vi "ClearAll.vi"(8 "Error In":errorcluster, 11 "CommunicationRefs":T1) -> (0 "error out":errorcluster)   [LabVIEW 2015]
uses:
  TypeDefs/CommunicationRefs.ctl
  TypeDefs/MessageCluster.ctl
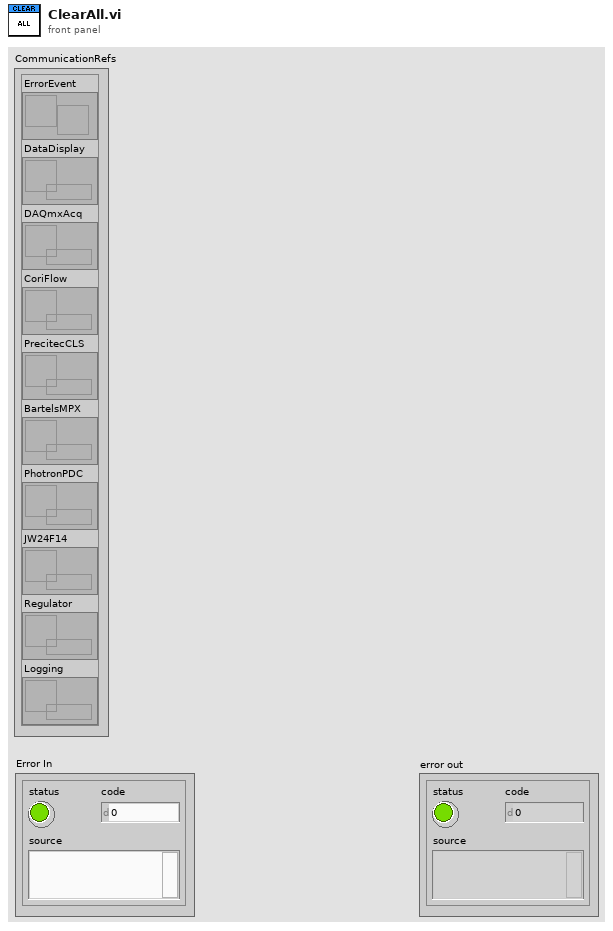
[diagram p1: front panel]
types:
  T1 = typedef "CommunicationRefs.ctl" = cluster{"ErrorEvent":refnum<user-event>, "DataDisplay":refnum<queue>, "DAQmxAcq":refnum<queue>, "CoriFlow":refnum<queue>, "PrecitecCLS":refnum<queue>, "BartelsMPX":refnum<queue>, "PhotronPDC":refnum<queue>, "JW24F14":refnum<queue>, "Regulator":refnum<queue>, "Logging":refnum<queue>}
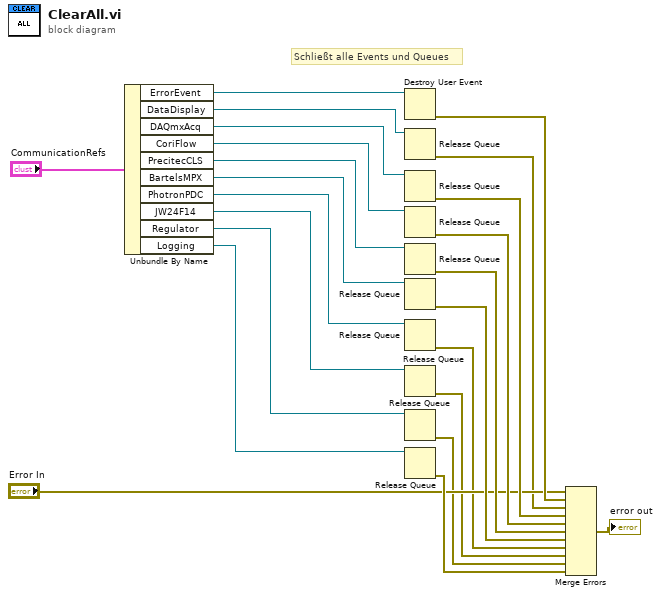
[diagram p0: block diagram]
diagram:
  # "Schließt alle Events und Queues"
  n1 = Unbundle By Name("CommunicationRefs") -> ("ErrorEvent"=w22:refnum<user-event>, "DataDisplay"=w8:refnum<queue>, "DAQmxAcq"=w20:refnum<queue>, "CoriFlow"=w19:refnum<queue>, "PrecitecCLS"=w18:refnum<queue>, "BartelsMPX"=w17:refnum<queue>, "PhotronPDC"=w5:refnum<queue>, "JW24F14"=w4:refnum<queue>, "Regulator"=w2:refnum<queue>, "Logging"=w16:refnum<queue>)
  n2 = Destroy User Event(user event=w22) -> (error out=w21:errorcluster)  [unwired: 1 in]
  n3 = Release Queue(queue=w8) -> (error out=w7:errorcluster)  [unwired: 2 in, 2 out]
  n4 = Release Queue(queue=w20) -> (error out=w15:errorcluster)  [unwired: 2 in, 2 out]
  n5 = Release Queue(queue=w19) -> (error out=w14:errorcluster)  [unwired: 2 in, 2 out]
  n6 = Release Queue(queue=w18) -> (error out=w13:errorcluster)  [unwired: 2 in, 2 out]
  n7 = Release Queue(queue=w17) -> (error out=w12:errorcluster)  [unwired: 2 in, 2 out]
  n8 = Release Queue(queue=w5) -> (error out=w6:errorcluster)  [unwired: 2 in, 2 out]
  n9 = Release Queue(queue=w4) -> (error out=w3:errorcluster)  [unwired: 2 in, 2 out]
  n10 = Release Queue(queue=w2) -> (error out=w1:errorcluster)  [unwired: 2 in, 2 out]
  n11 = Release Queue(queue=w16) -> (error out=w11:errorcluster)  [unwired: 2 in, 2 out]
  n12 = Merge Errors("Error In", w21, w7, w15, w14, w13, w12, w6, w3, w1, w11) -> (→"error out":errorcluster)
